vi "5-Cards.vi"() -> (0 "Array":i32[](array[numeric]), 1 "Array 2":i32[](array[numeric]))   [LabVIEW 2014]
panel:
  out "appended array 2":bool[](array[boolean])
  out "Numeric 2":i32
  out "Numeric":i32
  out "appended array":bool[](array[boolean])
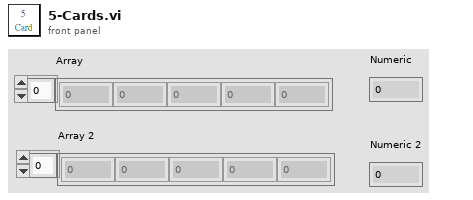
[diagram p1: front panel]
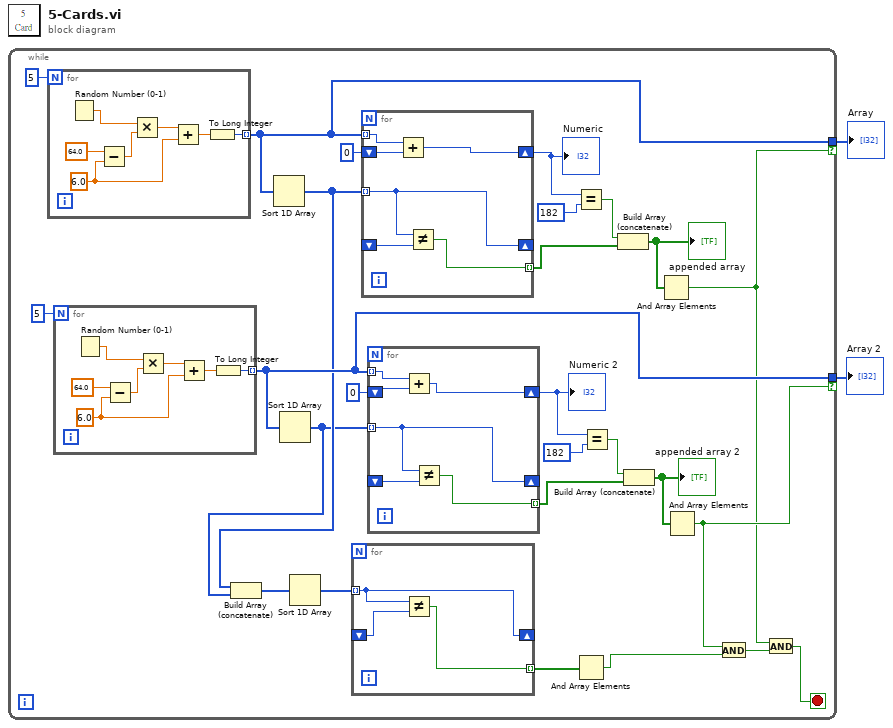
[diagram p0: block diagram]
diagram:
  n1 = while {
    tunnel: [w26] -> w2 if=w5
    tunnel: [w13] -> w1 if=w6
    stop <- w3 stop-if-true
    n2 = for {
      N: 5 -> [_]
      tunnel: [w51] -> w26 mode=indexing
      w53 = 6.0 ("y")
      n3 = Random Number (0-1)() -> (number: 0 to 1=w57:dbl)
      n4 = Subtract(x=64.0, y=w53) -> (x-y=w56:dbl)
      n5 = Multiply(x=w57, y=w56) -> (x*y=w54:dbl)
      n6 = Add(x=w54, y=w53) -> (x+y=w52:dbl)
      n7 = To Long Integer(number=w52) -> (32bit integer=w51:i32)
    }
    n8 = for {
      N: 5 -> [_]
      tunnel: [w38] -> w13 mode=indexing
      w40 = 6.0 ("y")
      n9 = Random Number (0-1)() -> (number: 0 to 1=w44:dbl)
      n10 = Subtract(x=64.0, y=w40) -> (x-y=w43:dbl)
      n11 = Multiply(x=w44, y=w43) -> (x*y=w41:dbl)
      n12 = Add(x=w41, y=w40) -> (x+y=w39:dbl)
      n13 = To Long Integer(number=w39) -> (32bit integer=w38:i32)
    }
    n14 = Sort 1D Array(array=w26) -> (sorted array=w12:i32[])
    n15 = Sort 1D Array(array=w13) -> (sorted array=w11:i32[])
    n16 = Build Array (concatenate)(w12, w11) -> (w10:i32[])
    n17 = Sort 1D Array(array=w10) -> (sorted array=w9:i32[])
    n18 = for {
      tunnel: w9 -> [w30] mode=indexing
      shift-right: [w30] -> _
      shift-left: _ -> [w31]
      tunnel: [w29] -> w8 mode=indexing
      n19 = Not Equal?(x=w30, y=w31) -> (x != y?=w29:bool)
    }
    n20 = for {
      tunnel: w26 -> [w48] mode=indexing
      shift-right: [w50] -> w22
      shift-left: 0 -> [w49]
      tunnel: w12 -> [w47] mode=indexing
      shift-right: [w47] -> _
      shift-left: _ -> [w46]
      tunnel: [w45] -> w25 mode=indexing
      n21 = Add(x=w48, y=w49) -> (x+y=w50:i32)
      n22 = Not Equal?(x=w47, y=w46) -> (x != y?=w45:bool)
    }
    "Numeric" <- w22
    n23 = for {
      tunnel: w13 -> [w35] mode=indexing
      shift-right: [w37] -> w19
      shift-left: 0 -> [w36]
      tunnel: w11 -> [w34] mode=indexing
      shift-right: [w34] -> _
      shift-left: _ -> [w33]
      tunnel: [w32] -> w16 mode=indexing
      n24 = Add(x=w35, y=w36) -> (x+y=w37:i32)
      n25 = Not Equal?(x=w34, y=w33) -> (x != y?=w32:bool)
    }
    "Numeric 2" <- w19
    n26 = Equal?(x=w22, y=182) -> (x = y?=w21:bool)
    n27 = And Array Elements(Boolean array=w8) -> (logical AND=w7:bool)
    n28 = Equal?(x=w19, y=182) -> (x = y?=w20:bool)
    n29 = Build Array (concatenate)(w21, w25) -> (w24:bool[])
    "appended array" <- w24
    n30 = Build Array (concatenate)(w20, w16) -> (w17:bool[])
    "appended array 2" <- w17
    n31 = And Array Elements(Boolean array=w24) -> (logical AND=w5:bool)
    n32 = And Array Elements(Boolean array=w17) -> (logical AND=w6:bool)
    n33 = And(x=w6, y=w7) -> (x .and. y?=w4:bool)
    n34 = And(x=w5, y=w4) -> (x .and. y?=w3:bool)
  }
  "Array" <- w2
  "Array 2" <- w1
